vi "DevDemo.vi"() -> ()   [LabVIEW 2012]
uses:
  Fun/Dev/SupportVi/DevState.ctl
  <vilib>/Instr/_visa.llb/VISA Configure Serial Port (Instr).vi
  Fun/Dev/DevControl.lvclass
panel:
  out "布尔":bool
  in  "‚€”µ":i32=10
  in  "数组 2":cluster{"裝置狀態":T1, "布尔":bool}[](array[cluster])
  in  "停止":bool
  in  "y":i32
  out "RX":string
  out "TX":string
  in  "VISA资源名称":refnum<visa-resource-name>
  out "数组":cluster{"Addr":u8, "裝置狀態":T1}[](array[cluster])
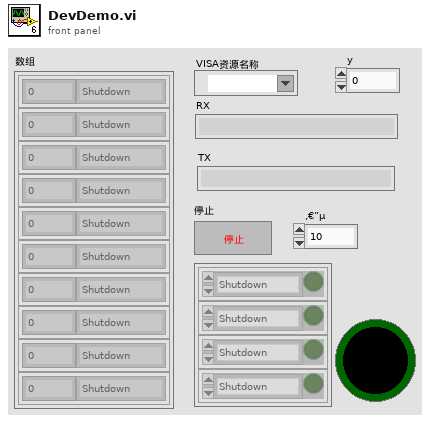
[diagram p1: front panel]
types:
  T1 = typedef "DevControl.lvclass/DevState.ctl" = enum16{"Shutdown", "PASS", "FAIL", "Idle", "Noresponse"}
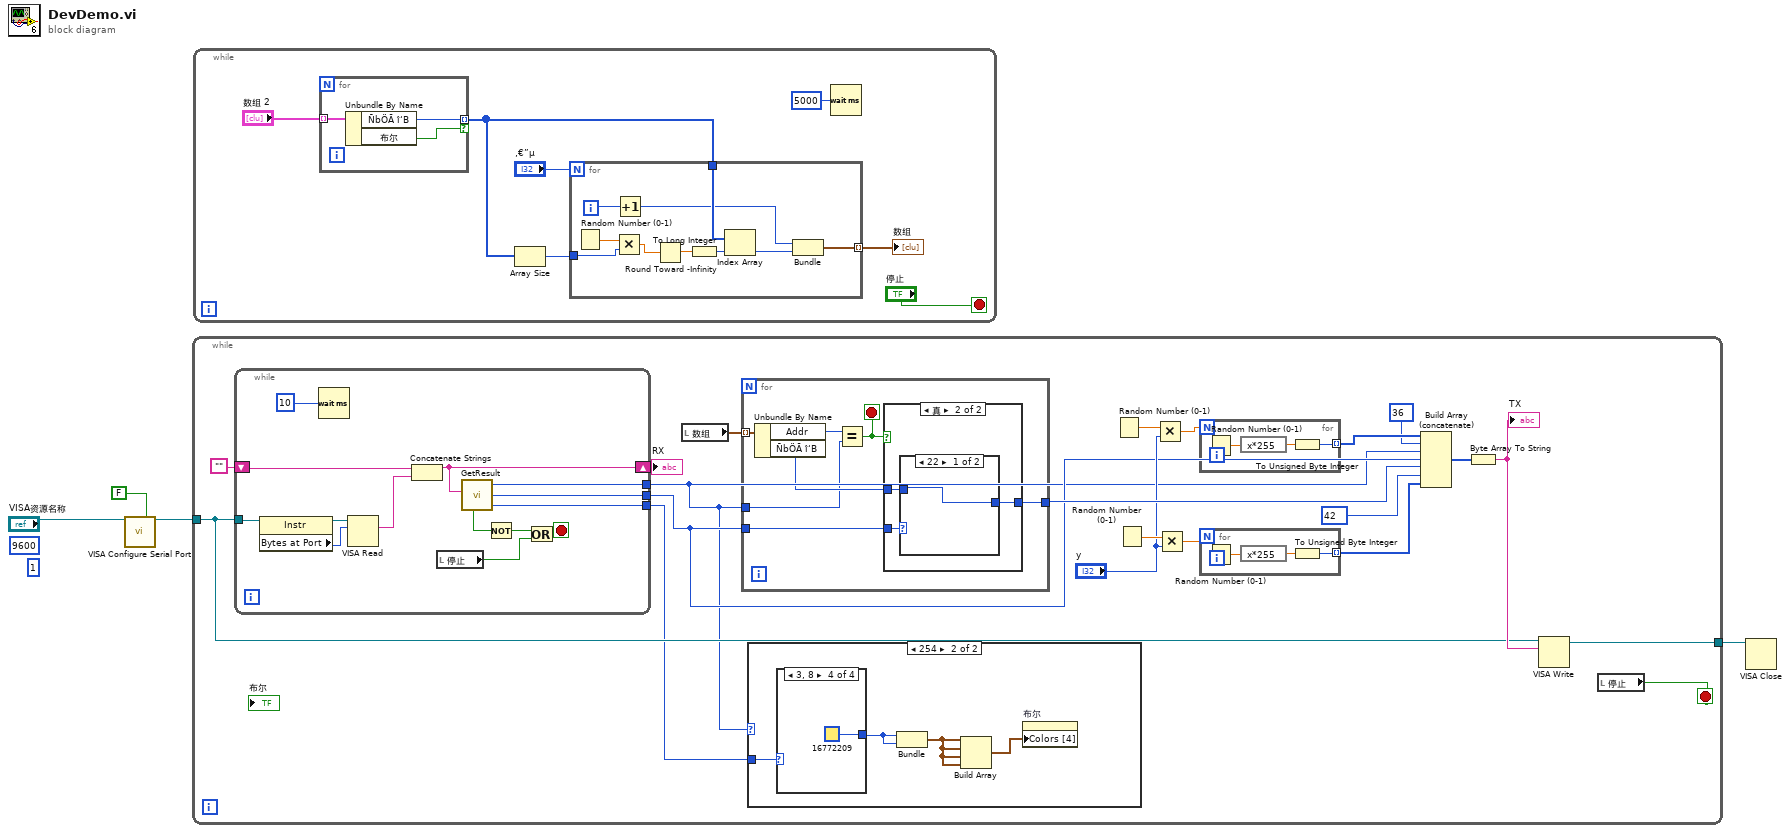
[diagram p0: block diagram]
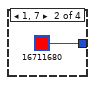
[diagram p4: hidden frame]
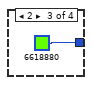
[diagram p5: hidden frame]
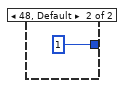
[diagram p7: hidden frame]
diagram:
  (unwired) 1 ("Retry")
  (unwired) u32 9600 ("波特率")
  n1 = call-poly "VISA Configure Serial Port"("VISA resource name"="VISA资源名称", "Enable Termination\nChar (T)"=FALSE ("Enable Termination\nChar (T)")) -> ("VISA resource name out"=w2:refnum<visa-resource-name>)  [unwired: 12 in, 1 out]
  n2 = while {
    tunnel: w2 -> [w9]
    tunnel: [w8] -> w1
    stop <- w12 stop-if-true
    n3 = while {
      shift-right: [w42] -> w11
      shift-left: "" -> [w45]
      tunnel: [w39] -> w6
      tunnel: [w38] -> w7
      tunnel: [w37] -> w5
      tunnel: w9 -> [w36]
      stop <- w44 stop-if-true
      n4 = property class="Instr"(reference=w36) -> (reference out=w35:refnum<visa-resource-name>, "Bytes at Port"=w34:u32)  [unwired: 1 in, 1 out]
      n5 = Wait (ms)(milliseconds to wait=10) -> ()  [unwired: 1 out]
      n6 = VISA Read(VISA resource name=w35, byte count=w34) -> (read buffer=w33:string)  [unwired: 1 in, 3 out]
      n7 = Concatenate Strings(w45, w33) -> (w42:string)
      n8 = local read "停止"() -> (w43:bool)
      n9 = call "GetResult.vi"("ReadBuff"=w42) -> ("Error?"=w40:bool, "Addr"=w39:u8, "Cmd"=w38:u8, "Data"=w37:u8)  [unwired: 4 in]
      n10 = Not(x=w40) -> (.not. x?=w41:bool)
      n11 = Or(x=w41, y=w43) -> (x .or. y?=w44:bool)
    }
    "RX" <- w11
    n12 = local read "数组"() -> (w25:cluster{"Addr":u8, "裝置狀態":T1}[])
    n13 = for {
      tunnel: w25 -> [w59] mode=indexing
      tunnel: [w57] -> w24
      tunnel: w6 -> [w54]
      tunnel: w7 -> [w53]
      stop <- w56 stop-if-true
      n14 = Unbundle By Name(w59) -> ("Addr"=w55:u8, "裝置狀態"=w58:T1)
      n15 = Equal?(x=w55, y=w54) -> (x = y?=w56:bool)
      n16 = case shown="真" w56 {
        tunnel: w53 -> [_ w62]
        tunnel: w58 -> [_ w61]
        tunnel: [_ w60] -> w57
        frame False {
        }
        frame True {
          n17 = case shown="22" w62 {
            tunnel: w61 -> [w63 _]
            tunnel: [w63 u8 1 ("Cmd")] -> w60
            frame 34 {
            }
            frame 48, Default {
            }
          }
        }
      }
    }
    n18 = case shown="254" w6 {
      tunnel: w5 -> [_ w29]
      frame 0, Default {
      }
      frame 254 {
        n19 = case shown="3, 8" w29 {
          tunnel: [_ u32 16711680 u32 6618880 u32 16772209] -> w28
          frame 0, Default {
          }
          frame 1, 7 {
          }
          frame 2 {
          }
          frame 3, 8 {
          }
        }
        n20 = Bundle(w28, w28) -> (w27:cluster{u32, u32})  [unwired: 1 in]
        n21 = Build Array(w27, w27, w27, w27) -> (w26:cluster{u32, u32}[])
        n22 = property on="布尔" class="Bool (严格)"("Colors [4]"=w26) -> ()  [unwired: 2 in, 2 out]
      }
    }
    n23 = Random Number (0-1)() -> (number: 0 to 1=w18:dbl)
    n24 = Random Number (0-1)() -> (number: 0 to 1=w17:dbl)
    n25 = Multiply(x=w18, y="y") -> (x*y=w16:dbl)
    n26 = Multiply(x=w17, y="y") -> (x*y=w15:dbl)
    n27 = for {
      N: w16 -> [_]
      tunnel: [w50] -> w23 mode=indexing
      n28 = Random Number (0-1)() -> (number: 0 to 1=w52:dbl)
      n29 = expression code="x*255"(w52) -> (w51:dbl)
      n30 = To Unsigned Byte Integer(number=w51) -> (unsigned 8bit integer=w50:u8)
    }
    n31 = for {
      N: w15 -> [_]
      tunnel: [w47] -> w20 mode=indexing
      n32 = Random Number (0-1)() -> (number: 0 to 1=w49:dbl)
      n33 = expression code="x*255"(w49) -> (w48:dbl)
      n34 = To Unsigned Byte Integer(number=w48) -> (unsigned 8bit integer=w47:u8)
    }
    n35 = Build Array (concatenate)(w23, 36, w6, w7, w24, 42, w20) -> (w19:i32[])
    n36 = Byte Array To String(unsigned byte array=w19) -> (string=w10:string)
    "TX" <- w10
    n37 = VISA Write(VISA resource name=w9, write buffer=w10) -> (VISA resource name out=w8:refnum<visa-resource-name>)  [unwired: 1 in, 2 out]
    n38 = local read "停止"() -> (w12:bool)
  }
  n39 = while {
    stop <- "停止" stop-if-true
    n40 = for {
      tunnel: "数组 2" -> [w74] mode=indexing
      tunnel: [w73] -> w65 mode=indexing if=w72
      n41 = Unbundle By Name(w74) -> ("裝置狀態"=w73:T1, "布尔"=w72:bool)
    }
    n42 = Array Size(array=w65) -> (size(s)=w66:i32)
    n43 = for {
      N: "‚€”µ" -> [_]
      tunnel: w65 -> [w82]
      tunnel: [w79] -> w70 mode=indexing
      tunnel: w66 -> [w77]
      i -> [w84]
      n44 = Random Number (0-1)() -> (number: 0 to 1=w78:dbl)
      n45 = Multiply(x=w78, y=w77) -> (x*y=w75:dbl)
      n46 = Increment(x=w84) -> (x+1=w80:i32)
      n47 = Round Toward -Infinity(1:w75) -> (0:w76:dbl)
      n48 = To Long Integer(number=w76) -> (32bit integer=w83:i32)
      n49 = Index Array(array=w82, index=w83) -> (element=w81:T1)
      n50 = Bundle(w80, "裝置狀態"=w81) -> (w79:cluster{i32, "裝置狀態":T1})  [unwired: 1 in]
    }
    "数组" <- w70
    n51 = Wait (ms)(milliseconds to wait=u32 5000 ("等待时间（毫秒）")) -> ()  [unwired: 1 out]
  }
  n52 = VISA Close(VISA resource name=w1) -> ()  [unwired: 1 in, 1 out]
